vi "upload-file.vi"(8 "error in (no error)":errorcluster, 9 "file":string, 10 "path":string, 11 "filepath":path) -> (0 "error out":errorcluster, 3 "filepath":string)   [LabVIEW 2015, in "lv-dropbox.lvlib" / "v2.lvlib"]
uses:
  v2.lvlib
  private/_controls/content_type.ctl
  _controls/error.ctl
  <vilib>/httpClient/POSTBuffer.vi
  <vilib>/httpClient/LabVIEWHTTPClient.lvlib
  lv-dropbox.lvlib
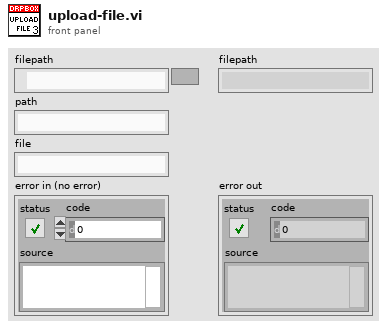
[diagram p1: front panel]
types:
  T1 = typedef "lv-dropbox.lvlib/content_type.ctl" = enum16{"<content_type>", "application/json", "application/octet-stream", "application/x-www-form-urlencoded"}
  T2 = typedef "lv-dropbox.lvlib/error.ctl" = enum16{"<error>", "file_too_big"}
  T3 = cluster{"name":string, "path_lower":string, "id":string, "client_modified":string, "server_modified":string, "rev":string, "size":u64}
  T4 = typedef "LabVIEWHTTPClient.lvlib/ClientHandle.ctl" = refnum<k1>
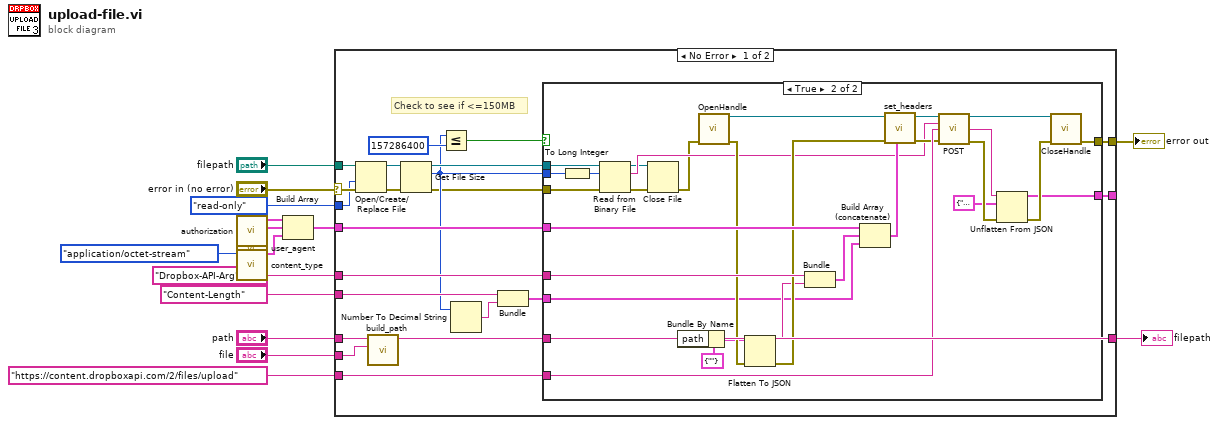
[diagram p0: block diagram]
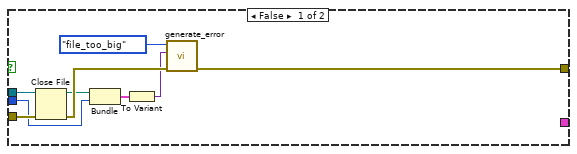
[diagram p2: hidden frame]
diagram:
  n1 = call "authorization.vi"() -> ("header"=w11:cluster{"header":string, "value":string})  [unwired: 11 in]
  n2 = call "user_agent.vi"() -> ("header"=w10:cluster{"header":string, "value":string})  [unwired: 11 in]
  n3 = call "content_type.vi"("content_type"=content_type."application/octet-stream") -> ("header"=w12:cluster{"header":string, "value":string})  [unwired: 10 in]
  n4 = Build Array(w11, w10, w12) -> (w6:cluster{"header":string, "value":string}[])
  n5 = case shown="No Error" "error in (no error)" {
    selector: "error in (no error)" -> [w36 w76]
    tunnel: "path" -> [w17 _]
    tunnel: enum16{"read/write", "read-only", "write-only"}."read-only" ("access (0:read/write)") -> [w35 _]
    tunnel: "Dropbox-API-Arg" ("header") -> [w34 _]
    tunnel: "Content-Length" ("header") -> [w33 _]
    tunnel: w6 -> [w32 _]
    tunnel: "https://content.dropboxapi.com/2/files/upload" ("url") -> [w31 _]
    tunnel: [w30 w76] -> w4
    tunnel: "filepath" -> [w22 _]
    tunnel: [w19 _] -> _
    tunnel: "file" -> [w18 _]
    tunnel: [w16 _] -> w1
    frame No Error {
      # "Check to see if <=150MB"
      n6 = Open/Create/Replace File(file path (use dialog)=w22, error in=w36, access (0:read/write)=w35) -> (refnum out=w21:refnum<file>, error out=w26:errorcluster)  [unwired: 3 in, 1 out]
      n7 = call "build_path.vi"("path"=w18, "base_path"=w17) -> ("path"=w16:string)  [unwired: 9 in]
      n8 = Get File Size(file=w21, error in=w26) -> (refnum out=w25:refnum<file>, size (in bytes)=w24:i64, 0:w23:errorcluster)
      n9 = Less Or Equal?(x=w24, y=i64 157286400) -> (x <= y?=w20:bool)
      n10 = Number To Decimal String(number=w24) -> (decimal integer string=w28:string)  [unwired: 1 in]
      n11 = Bundle("header"=w33, w28) -> (w27:cluster{"header":string, string})  [unwired: 1 in]
      n12 = case shown="True" w20 {
        tunnel: w16 -> [_ w75]
        tunnel: w34 -> [_ w74]
        tunnel: w32 -> [_ w73]
        tunnel: w31 -> [_ w72]
        tunnel: [w44 w71] -> w30
        tunnel: w27 -> [_ w56]
        tunnel: w25 -> [w42 w53]
        tunnel: w24 -> [w39 w52]
        tunnel: w23 -> [w43 w50]
        tunnel: [_ w46] -> w19
        frame False {
          n13 = Close File(refnum=w42, error in=w43) -> (path=w40:path, error out=w41:errorcluster)
          n14 = Bundle("path"=w40, "size (in bytes)"=w39) -> (w38:cluster{"path":path, "size (in bytes)":i64})  [unwired: 1 in]
          n15 = To Variant(anything=w38) -> (Variant=w37:variant)
          n16 = call "generate_error.vi"("error in (no error)"=w41, "data"=w37, "error"=error."file_too_big") -> ("error out"=w44:errorcluster)  [unwired: 8 in]
        }
        frame True {
          n17 = To Long Integer(number=w52) -> (32bit integer=w51:i32)
          n18 = Read from Binary File(8:w50, 10:w51, 11:w53) -> (0:w48:errorcluster, 2:w54:string, 3:w49:refnum<file>)  [unwired: 3 in, 1 out]
          n19 = Close File(refnum=w49, error in=w48) -> (error out=w47:errorcluster)  [unwired: 1 out]
          n20 = Bundle By Name(cluster=cluster{"path":string} {"path"=""}, "path"=w75) -> (w64:cluster{"path":string})
          n21 = call <vilib>:"OpenHandle.vi"("error in (no error)"=w47) -> ("client handle out"=w61:T4, "error out"=w68:errorcluster)  [unwired: 13 in]
          n22 = Flatten To JSON(anything=w64, error in (no error)=w68) -> (JSON string=w60:string, 11:w67:errorcluster)  [unwired: 1 in]
          n23 = Bundle("header"=w74, "JSON string"=w60) -> (w57:cluster{"header":string, "JSON string":string})  [unwired: 1 in]
          n24 = Build Array (concatenate)(w73, w57, w56) -> (w55:cluster{"header":string, "JSON string":string}[])
          n25 = call "set_headers.vi"("header_value []"=w55, "error in (no error)"=w67, "client_handle in"=w61) -> ("error out"=w58:errorcluster, "client_handle out"=w59:T4)  [unwired: 7 in]
          n26 = call-poly <vilib>:"POST.vi"("client handle"=w59, "url"=w54, "buffer"=w72, "error in (no error)"=w58) -> ("client handle out"=w63:T4, "body"=w66:string, "error out"=w70:errorcluster)  [unwired: 8 in, 1 out]
          n27 = Unflatten From JSON(JSON string=w66, type and defaults=T3 {"name"="", "path_lower"="", "id"="", "client_modified"="", "server_modified"="", "rev"="", "size"=0}, error in (no error)=w70) -> (value=w46:T3, error out=w69:errorcluster)  [unwired: 4 in]
          n28 = call <vilib>:"CloseHandle.vi"("client handle"=w63, "error in (no error)"=w69) -> ("error out"=w71:errorcluster)  [unwired: 13 in]
        }
      }
    }
    frame Error {
    }
  }
  "error out" <- w4
  "filepath" <- w1
